vi "Cross_Corr_Large_slip.vi"() -> (5 "Plug in titles":string[](array[string]), 7 "Plug in values":string[](array[string]))   [LabVIEW 2010]
uses:
  Controls/Post_Process.ctl
  Globals/Meas_global.vi
  Globals/Plug_in_data_global.vi
  <vilib>/Analysis/NI_AALBase.lvlib
panel:
  in  "Auto guess slip":bool
  out "Slippage(ms)":dbl
  out "Waveform Graph":cluster{dbl, "Delta Slip":dbl, dbl[]}(graph)
  in  "No of steps":i32=200
  in  "Delta Slip":dbl=2.0 format="%.2f"
  out "Correlation coefficient":dbl
  in  "Approx Slip (ms)":dbl format="%.2f"
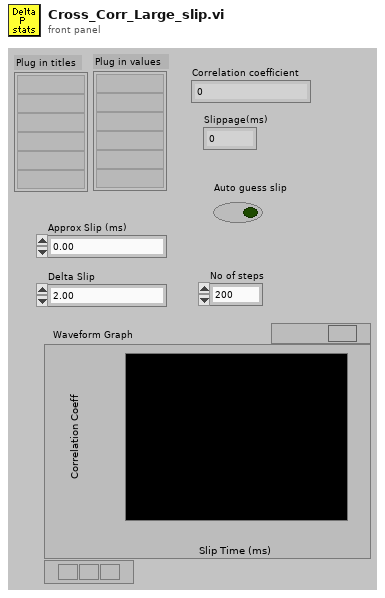
[diagram p1: front panel]
types:
  T1 = typedef "Post_Process.ctl" = enum16{"Take New Data", "Post Process Raw Data File"}
  T2 = cluster{"Name":string, "X":dbl, "Y":dbl, "Z":dbl}[]
  T3 = cluster{"Name":string, "X":dbl, "Y":dbl, "Z":dbl}
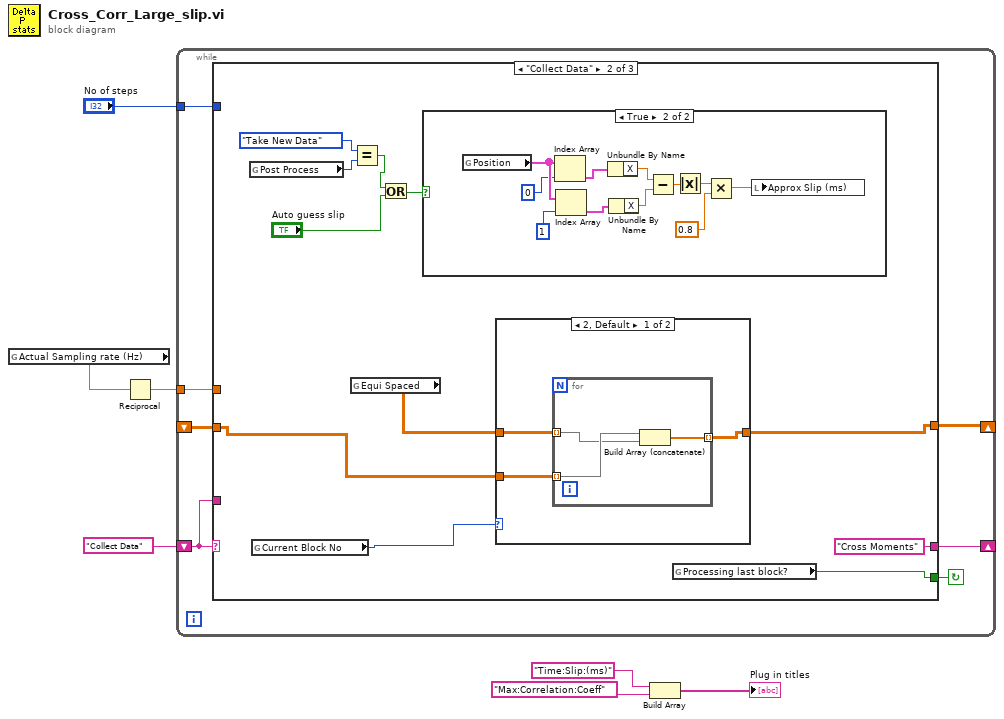
[diagram p0: block diagram]
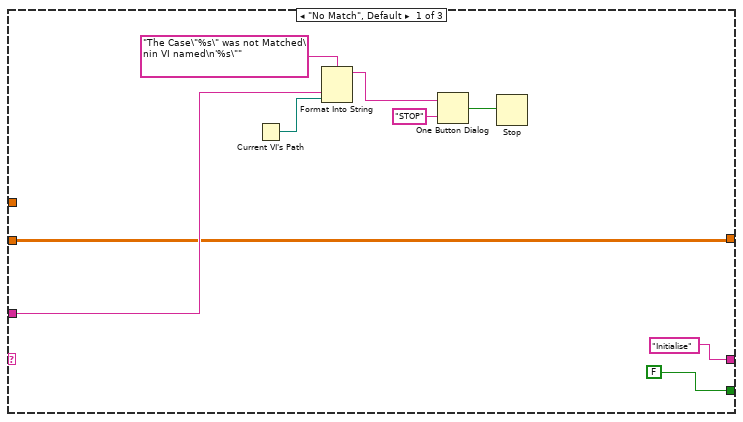
[diagram p2: hidden frame]
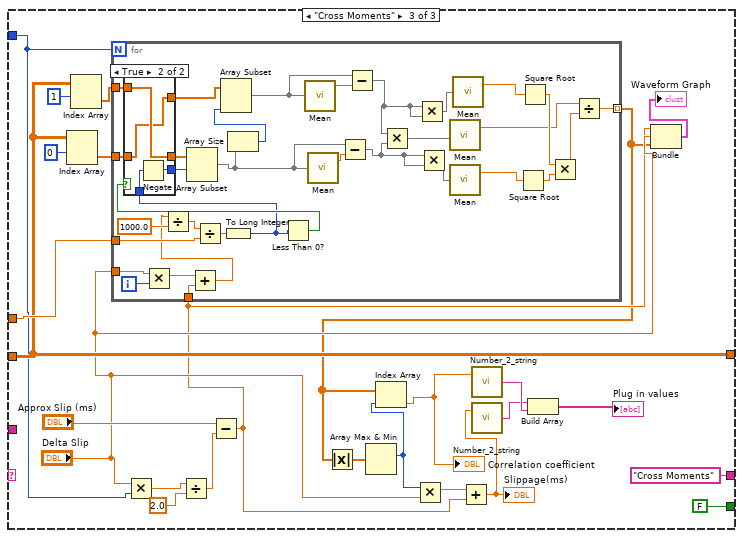
[diagram p5: hidden frame]
diagram:
  n1 = global read "Meas_global.vi" "Actual Sampling rate (Hz)"() -> (w5:dbl)
  n2 = Reciprocal(x=w5) -> (1/x=w6:dbl)
  n3 = while {
    shift-left: "Collect Data" -> [w12]
    shift-right: [w13] -> _
    tunnel: w6 -> [w11]
    shift-right: [w10] -> _
    shift-left: _ -> [w9]
    tunnel: "No of steps" -> [w8]
    stop <- w14 continue-if-true
    n4 = case shown="\"Collect Data\"" w12 {
      tunnel: [FALSE w29 FALSE] -> w14
      tunnel: ["Initialise" "Cross Moments" "Cross Moments"] -> w13
      tunnel: w12 -> [w18 _ _]
      tunnel: w11 -> [_ _ w73]
      tunnel: [w15 w32 w71] -> w10
      tunnel: w9 -> [w15 w31 w71]
      tunnel: w8 -> [_ _ w65]
      frame "No Match", Default {
        n5 = Current VI's Path() -> (path=w17:path)
        n6 = Format Into String(format string="The Case\"%s\" was not Matched\nin VI named\n'%s\"" ("Format String"), w18, w17) -> (resulting string=w21:string)  [unwired: 2 in, 1 out]
        n7 = One Button Dialog(message=w21, button name ("OK")="STOP") -> (true=w19:bool)
        n8 = Stop(stop? (T)=w19) -> ()
      }
      frame "Collect Data" {
        n9 = global read "Meas_global.vi" "Post Process"() -> (w28:T1)
        n10 = global read "Meas_global.vi" "Current Block No"() -> (w33:i32)
        n11 = global read "Plug_in_data_global.vi" "Equi Spaced"() -> (w30:dbl[][])
        n12 = Equal?(x=Post_Process."Take New Data" ("Post Process"), y=w28) -> (x = y?=w26:bool)
        n13 = Or(x=w26, y="Auto guess slip") -> (x .or. y?=w24:bool)
        n14 = case shown="True" w24 {
          frame False {
          }
          frame True {
            n15 = global read "Meas_global.vi" "Position"() -> (w45:T2)
            n16 = Index Array(array=w45, index=0) -> (element=w41:T3)
            n17 = Index Array(array=w45, index=1) -> (element=w42:T3)
            n18 = Unbundle By Name(w41) -> ("X"=w40:dbl)
            n19 = Unbundle By Name(w42) -> ("X"=w39:dbl)
            n20 = Subtract(x=w40, y=w39) -> (x-y=w38:dbl)
            n21 = Absolute Value(x=w38) -> (abs(x)=w37:dbl)
            n22 = Multiply(x=w37, y=0.8) -> (x*y=w36:dbl)
            n23 = local write "Approx Slip (ms)"(w36) -> ()
          }
        }
        n24 = case shown="2, Default" w33 {
          tunnel: [w46 w52] -> w32
          tunnel: w30 -> [w47 w52]
          tunnel: w31 -> [w48 _]
          frame 2, Default {
            n25 = for {
              tunnel: w48 -> [w51] mode=indexing
              tunnel: w47 -> [w50] mode=indexing
              tunnel: [w49] -> w46 mode=indexing
              n26 = Build Array (concatenate)(w51, w50) -> (w49:dbl[])
            }
          }
          frame 1 {
          }
        }
        n27 = global read "Meas_global.vi" "Processing last block?"() -> (w29:bool)
      }
      frame "Cross Moments" {
        n28 = Index Array(array=w71, index (row)=0) -> (element=w72:dbl[])  [unwired: 1 in]
        n29 = Index Array(array=w71, index (row)=1) -> (element=w70:dbl[])  [unwired: 1 in]
        n30 = Multiply(x="Delta Slip", y=w65) -> (x*y=w69:dbl)
        n31 = Divide(x=w69, y=2.0) -> (x/y=w66:dbl)
        n32 = Subtract(x="Approx Slip (ms)", y=w66) -> (x-y=w61:dbl)
        n33 = for {
          N: w65 -> [_]
          tunnel: w73 -> [w108]
          tunnel: w72 -> [w80]
          tunnel: w70 -> [w82]
          tunnel: "Delta Slip" -> [w90]
          tunnel: w61 -> [w88]
          tunnel: [w86] -> w54 mode=indexing
          i -> [w91]
          n34 = Multiply(x=w90, y=w91) -> (x*y=w89:dbl)
          n35 = Add(x=w89, y=w88) -> (x+y=w87:dbl)
          n36 = Divide(x=w87, y=1000.0) -> (x/y=w109:dbl)
          n37 = Divide(x=w109, y=w108) -> (x/y=w85:dbl)
          n38 = To Long Integer(number=w85) -> (32bit integer=w78:i32)
          n39 = Less Than 0?(x=w78) -> (x < 0?=w84:bool)
          n40 = case shown="True" w84 {
            tunnel: [w112 w117] -> w83
            tunnel: w82 -> [w113 w117]
            tunnel: [w113 w116] -> w81
            tunnel: w80 -> [w112 w116]
            tunnel: [w111 w114] -> w79
            tunnel: w78 -> [w111 w115]
            frame False {
            }
            frame True {
              n41 = Negate(x=w115) -> (-x=w114:i32)
            }
          }
          n42 = Array Subset(array=w83, index=w79) -> (w94:dbl[])  [unwired: 1 in]
          n43 = Array Size(array=w94) -> (size(s)=w107:i32)
          n44 = Array Subset(array=w81, length=w107) -> (w97:dbl[])  [unwired: 1 in]
          n45 = call <vilib>:"Mean.vi"("X"=w97) -> ("mean"=w96:dbl)  [unwired: 1 out]
          n46 = call <vilib>:"Mean.vi"("X"=w94) -> ("mean"=w95:dbl)  [unwired: 1 out]
          n47 = Subtract(x=w94, y=w95) -> (x-y=w93:dbl[])
          n48 = Subtract(x=w97, y=w96) -> (x-y=w92:dbl[])
          n49 = Multiply(x=w92, y=w93) -> (x*y=w106:dbl[])
          n50 = Multiply(x=w92, y=w92) -> (x*y=w104:dbl[])
          n51 = Multiply(x=w93, y=w93) -> (x*y=w105:dbl[])
          n52 = call <vilib>:"Mean.vi"("X"=w106) -> ("mean"=w99:dbl)  [unwired: 1 out]
          n53 = call <vilib>:"Mean.vi"("X"=w105) -> ("mean"=w103:dbl)  [unwired: 1 out]
          n54 = call <vilib>:"Mean.vi"("X"=w104) -> ("mean"=w102:dbl)  [unwired: 1 out]
          n55 = Square Root(x=w103) -> (sqrt(x)=w100:dbl)
          n56 = Square Root(x=w102) -> (sqrt(x)=w101:dbl)
          n57 = Multiply(x=w101, y=w100) -> (x*y=w98:dbl)
          n58 = Divide(x=w99, y=w98) -> (x/y=w86:dbl)
        }
        n59 = Absolute Value(x=w54) -> (abs(x)=w56:dbl[])
        n60 = Array Max & Min(array=w56) -> (max index (indices)=w55:i32)  [unwired: 3 out]
        n61 = Index Array(array=w54, index=w55) -> (element=w53:dbl)
        "Correlation coefficient" <- w53
        n62 = Multiply(x=w55, y="Delta Slip") -> (x*y=w63:dbl)
        n63 = Add(x=w63, y=w61) -> (x+y=w60:dbl)
        "Slippage(ms)" <- w60
        n64 = call "Number_2_string.vi"("number"=w53) -> ("String"=w59:string)  [unwired: 1 in]
        n65 = call "Number_2_string.vi"("number"=w60) -> ("String"=w58:string)  [unwired: 1 in]
        n66 = Build Array(w58, w59) -> (→"Plug in values":string[])
        n67 = Bundle(w61, "Delta Slip"="Delta Slip", w54) -> (→"Waveform Graph":cluster{dbl, "Delta Slip":dbl, dbl[]})  [unwired: 1 out]
      }
    }
  }
  n68 = Build Array("Time:Slip:(ms)" ("element"), "Max:Correlation:Coeff" ("element")) -> (→"Plug in titles":string[])
